vi "Double Value to String.vi"(10 "Value":dbl caption="数值") -> (2 "String":string caption="字符串")   [LabVIEW 2023, in "Longer Pump dLSP501 Series.lvlib"]
uses:
  <instrlib>/Longer Pump dLSP501 Modbus RTU Series/Longer Pump dLSP501 Series.lvlib
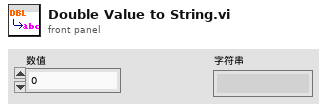
[diagram p1: front panel]
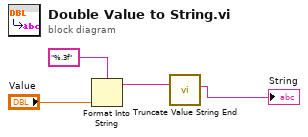
[diagram p0: block diagram]
diagram:
  n1 = Format Into String(format string="%.3f", "Value") -> (resulting string=w2:string)  [unwired: 2 in, 1 out]
  n2 = call <instrlib>:"Truncate Value String End.vi"("Value String In"=w2) -> ("Value String Out"=→"String":string)  [unwired: 10 in]
